vi "HELP.vi"() -> ()   [LabVIEW 2014]
panel:
  in  "确定":bool
  out "说明":string
  # "欢迎使用稻草人测控系统"
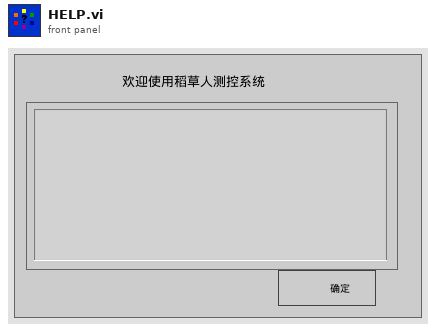
[diagram p1: front panel]
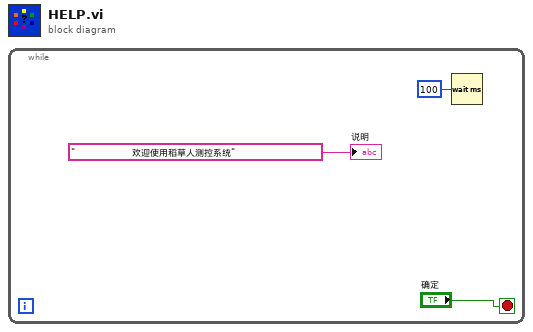
[diagram p0: block diagram]
diagram:
  n1 = while {
    stop <- "确定" stop-if-true
    n2 = Wait (ms)(milliseconds to wait=u32 100 ("等待时间（毫秒）")) -> ()  [unwired: 1 out]
    "说明" <- "                   欢迎使用稻草人测控系统" ("说明")
  }
